vi "runWholeDirectory.vi"(8 "error in (no error)":errorcluster, 11 "ExperimentRunner in":refnum<class "ExperimentRunner.lvclass">) -> (0 "error out":errorcluster, 3 "ExperimentRunner out":refnum<class "ExperimentRunner.lvclass">)   [LabVIEW 2011, in "Views.lvlib" / "ExperimentControl.lvlib" / "ExperimentRunner.lvclass"]
doc: "Run the whole script list."
uses:
  ExperimentRunner.lvclass
panel:
  in  "status in":refnum<vi>
  out "status out":refnum<vi>
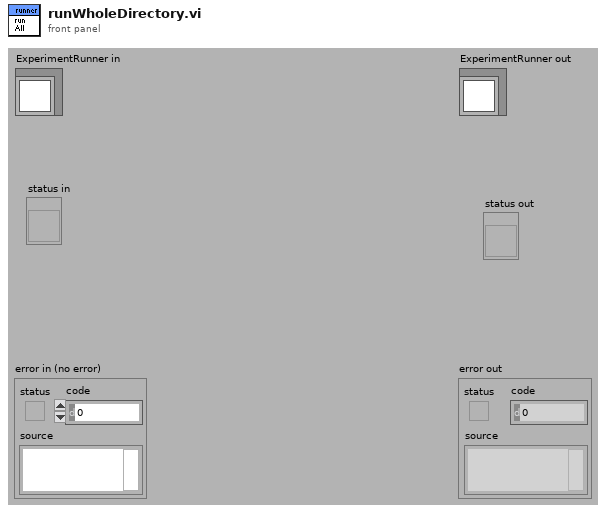
[diagram p1: front panel]
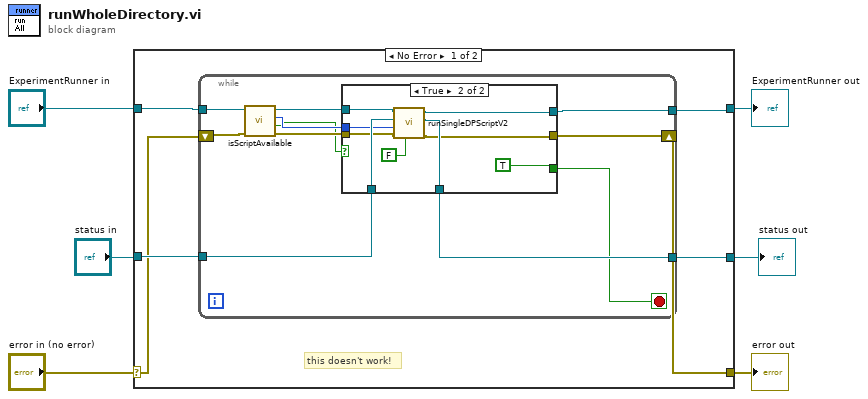
[diagram p0: block diagram]
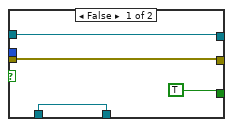
[diagram p2: hidden frame]
diagram:
  n1 = case shown="No Error" "error in (no error)" {
    selector: "error in (no error)" -> [w9 w38]
    tunnel: [w8 w38] -> w5
    tunnel: [w10 w37] -> w3
    tunnel: "ExperimentRunner in" -> [w7 w37]
    tunnel: "status in" -> [w12 _]
    tunnel: [w11 _] -> w2
    frame No Error {
      # "this doesn't work!"
      n2 = while {
        tunnel: w12 -> [w23]
        tunnel: [w22] -> w11
        tunnel: [w21] -> w10
        tunnel: w7 -> [w19]
        shift-right: [w20] -> w8
        shift-left: w9 -> [w17]
        stop <- w13 stop-if-true
        n3 = call "isScriptAvailable.vi"("error in (no error)"=w17, "ExperimentRunner in"=w19) -> ("error out"=w16:errorcluster, "available"=w14:bool, "selectedScript"=w15:i32, "ExperimentRunner out"=w18:refnum<class "ExperimentRunner.lvclass">)  [unwired: 6 in]
        n4 = case shown="True" w14 {
          tunnel: w23 -> [w25 w32]
          tunnel: [w25 w33] -> w22
          tunnel: [w27 w34] -> w21
          tunnel: [w26 w29] -> w20
          tunnel: w18 -> [w27 w35]
          tunnel: w16 -> [w26 w30]
          tunnel: w15 -> [_ w31]
          tunnel: [TRUE TRUE] -> w13
          frame False {
          }
          frame True {
            n5 = call "runSingleDPScriptV2.vi"("HWLoop?"=FALSE, "error in (no error)"=w30, "index"=w31, "status in"=w32, "ExperimentRunner in"=w35) -> ("error out"=w29:errorcluster, "status out"=w33:refnum<vi>, "ExperimentRunner out"=w34:refnum<class "ExperimentRunner.lvclass">)  [unwired: 4 in]
          }
        }
      }
    }
    frame Error {
    }
  }
  "error out" <- w5
  "ExperimentRunner out" <- w3
  "status out" <- w2
